vi "Sample Panel.vi"(8 "error in (no error)":errorcluster, 9 "L_Or_R":string, 10 "Measure_No":i64, 11 "connection reference":T1) -> (0 "error out":errorcluster)   [LabVIEW 2015, in "Sample.lvlib"]
uses:
  Sample.lvlib
  <vilib>/userdefined/High Color/IMAQdx.ctl
  Sub VIs/DAQ/DAQ.lvlib
  Sub VIs/CCD/CCD.lvlib
  Sub VIs/Database Processing/Database Processing.lvlib
  <vilib>/addons/database/NI_Database_API.lvlib
  <vilib>/addons/database/_DB Variant To Data/Database Variant To Data.xnode
  Sub VIs/Database Processing/Support/Table/Biometry.ctl
  support/User Event - Stop/User Event - Stop.lvlib
  support/Message Queue/Message Queue.lvlib
  support/Message Queue/Enqueue Message (Single).vi
  Sub VIs/DAQ/DAQ Configuration.ctl
  Sub VIs/CCD/Support/CCD Configuration.ctl
  Support/Sample Configuration.ctl
  <vilib>/Analysis/3filter.llb/Filter Passband Type.ctl
  <vilib>/Analysis/NI_AALBase.lvlib
  <vilib>/Analysis/4window.llb/windowTd.ctl
  <vilib>/Analysis/NI_AALPro.lvlib
  Sub VIs/Digital Signal Processing/Support/DSP Configuration.ctl
  Sub VIs/Digital Signal Processing/Digital Signal Processing.lvlib
  <vilib>/vision/Image Controls.llb/IMAQ Image.ctl
  <vilib>/addons/database/Connection.llb/Conn ObjectReference.ctl
panel:
  in  "Sample":bool
  out "Asan Signal":dbl[](graph)
  in  "停止":bool
  out "CCD Image":T2(plugin-control)
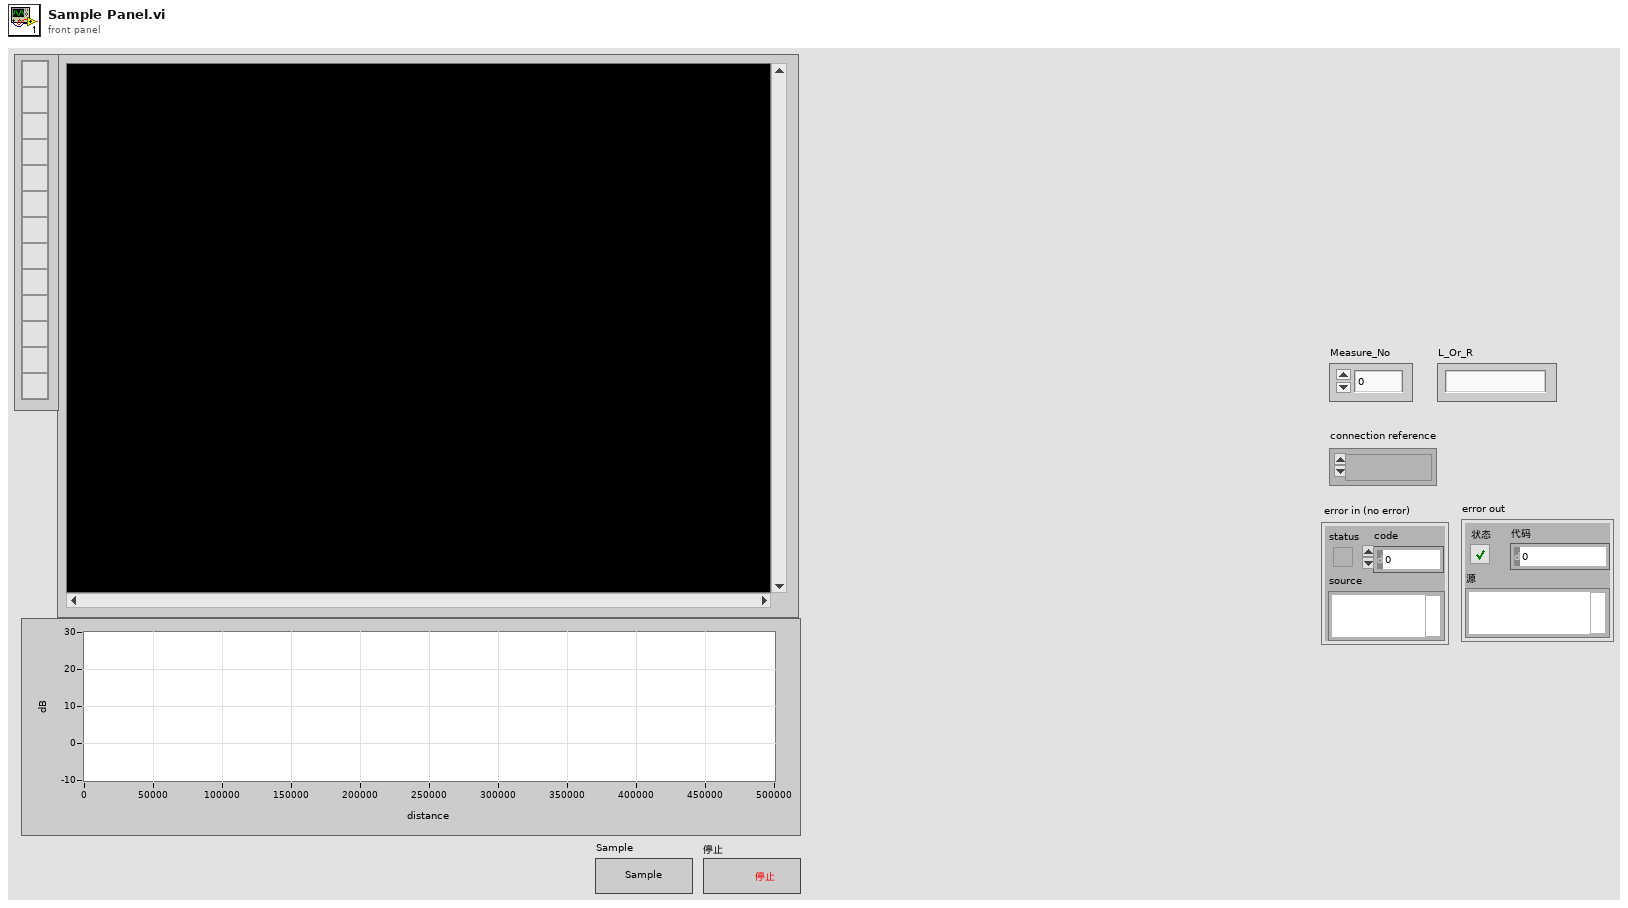
[diagram p1: front panel]
types:
  T1 = typedef "NI_Database_API.lvlib/Conn ObjectReference.ctl" = refnum<k1>
  T2 = typedef "IMAQ Image.ctl" = refnum<image>
  T3 = typedef "Biometry.ctl" = cluster{"Measure_ID":i64, "Measure_No":i64, "Ordinal":i64, "L_Or_R":string, "CCT":sgl, "CCT__State":string, "ACD":sgl, "ACD__State":string, "LT":sgl, "LT__State":string, "RT":sgl, "RT__State":string, "AL":sgl, "AL__State":string, "PD":sgl, "PD__State":string, "PCX":sgl, "PCY":sgl, "WTW":sgl, "WTW__State":string, "ICX":sgl, "ICY":sgl, "K_flat":sgl, "K_steep":sgl, "K_AST":sgl, "K__State":string, "Ascan_data_Original":string, "picture_pupil_Original":string, "picture_WTW_Original":string, "Ascan_data_Processing":string, "picture_pupil_Processing":string, "picture_WTW_Processing":string, "picture_Processing_K":string, "picture_Processing_ALL":string}
  T4 = typedef "Digital Signal Processing.lvlib/DSP Configuration.ctl" = cluster{"Sampling Frequency":dbl, "filter type":T5, "RF Filter Low Frequency":dbl, "RF Filter High Frequency":dbl, "RF Filter Taps":i32, "window":T6, "RF window parameter":dbl, "filter type 2":T5, "Demodulated Filter Low Frequency":dbl, "Demodulated Filter HighFrequency":dbl, "Demodulated Filter Order":i32, "SPAN":i32, "Logarithmic Base":dbl, "Noise path":string, "Work position parameter":i32[]}
  T5 = typedef "NI_AALBase.lvlib/Filter Passband Type.ctl" = enum32{"Lowpass", "Highpass", "Bandpass", "Bandstop"}
  T6 = typedef "NI_AALPro.lvlib/windowTd.ctl" = u32
  T7 = typedef "Sample.lvlib/Sample Configuration.ctl" = cluster{"DAQ Configuration":T8, "CCD Configuration":T9, "DSP Parameter":T4}
  T8 = typedef "DAQ.lvlib/DAQ Configuration.ctl" = cluster{"hDevice":i32, "DevNum":u8, "Configuration Parameter":i32[], "READ_MAX_LEN":i32, "DO":bool[]}
  T9 = typedef "CCD.lvlib/CCD Configuration.ctl" = cluster{"Session In":T10, "New Image":T2}
  T10 = typedef "IMAQdx.ctl" = refnum<k21>
  T11 = typedef "Message Queue.lvlib/All Message Queues Sample Panel.ctl" = cluster{"UI":refnum<queue>, "CAM":refnum<queue>, "CAM Log":refnum<queue>, "DAQ":refnum<queue>, "DSP":refnum<queue>, "DAQ Log":refnum<queue>, "DAQ Read Digital":refnum<queue>}
  T12 = cluster{"filter structure":enum32{"IIR 2nd Order", "IIR 4th Order"}, "Reverse Coefficients":dbl[], "Forward Coefficients":dbl[]}
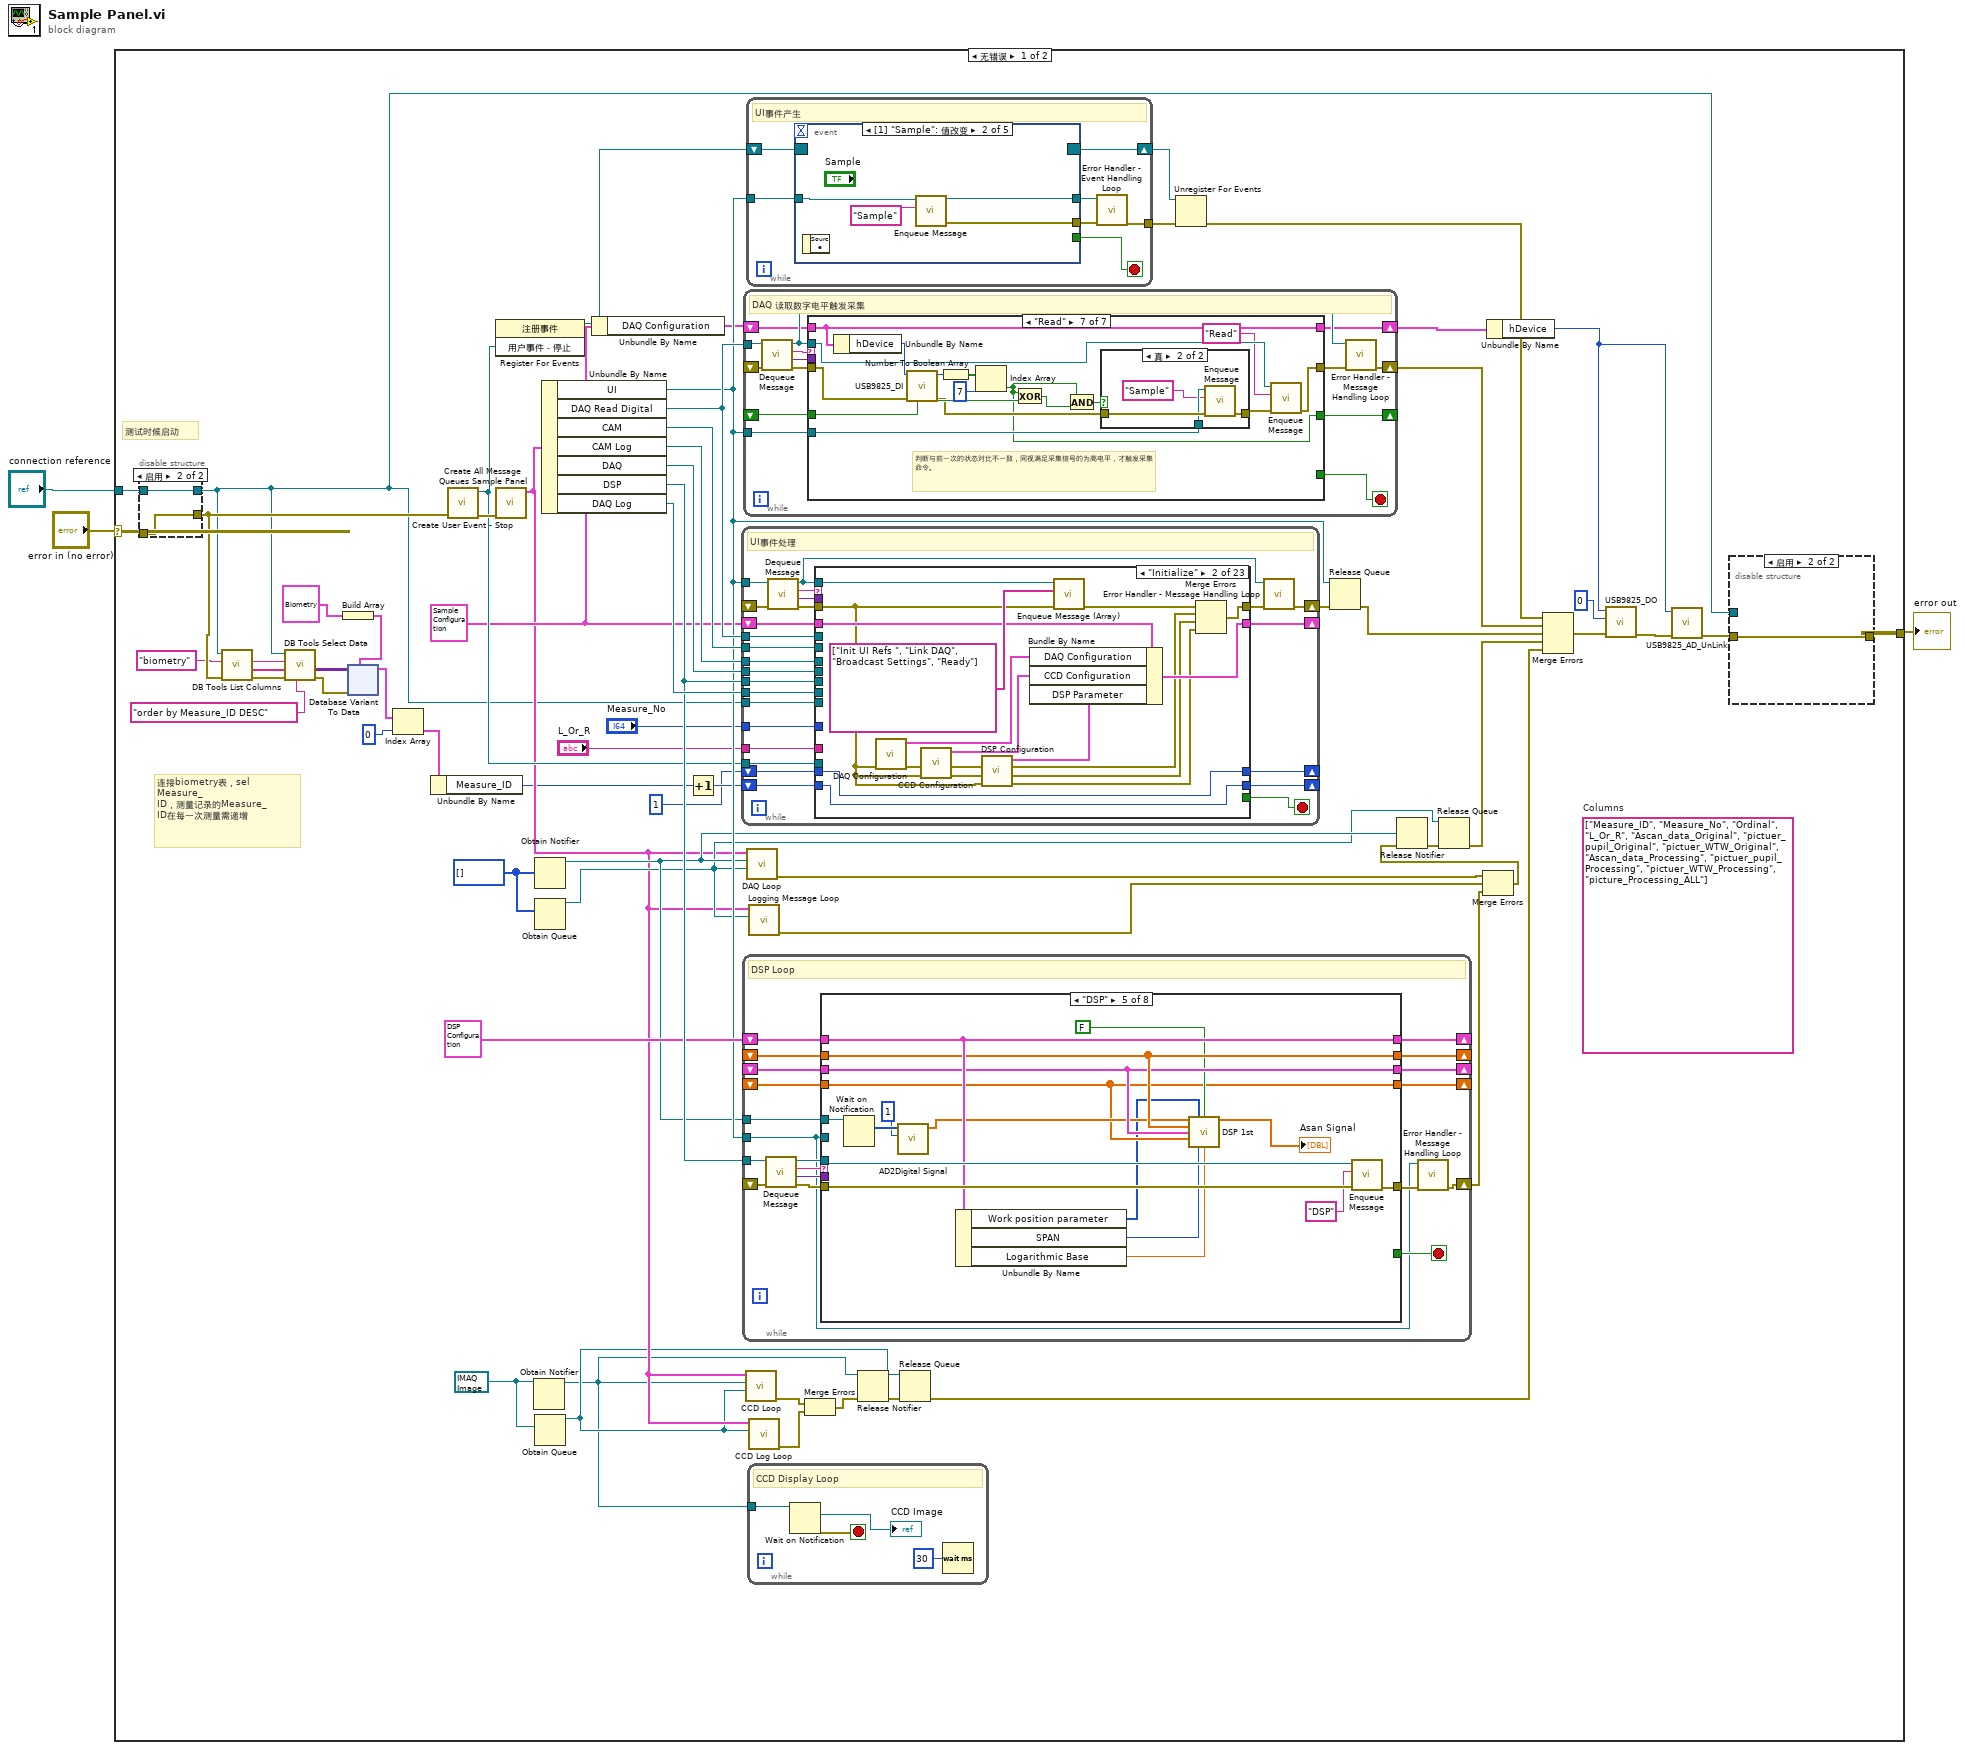
[diagram p0: block diagram]
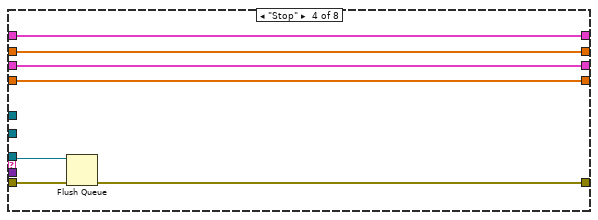
[diagram p5: hidden frame]
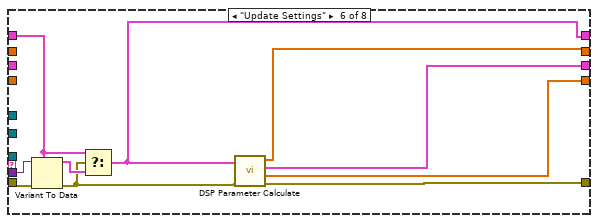
[diagram p6: hidden frame]
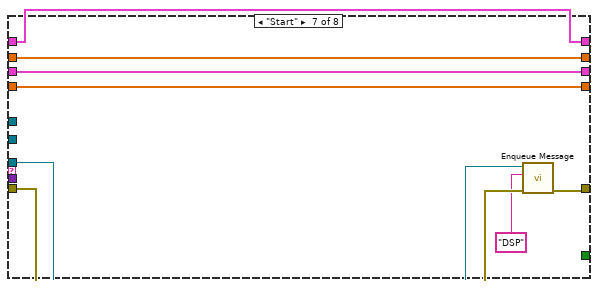
[diagram p7: hidden frame]
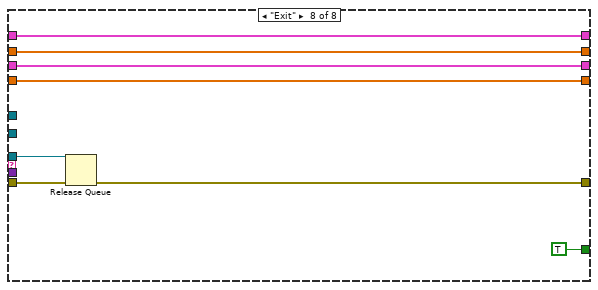
[diagram p8: hidden frame]
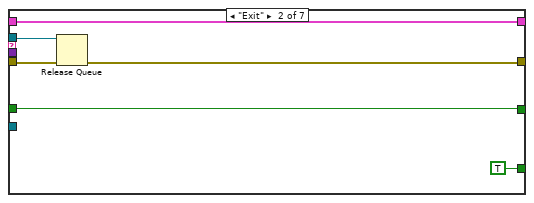
[diagram p10: hidden frame]
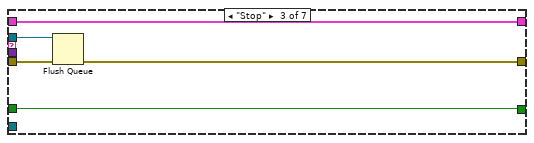
[diagram p11: hidden frame]
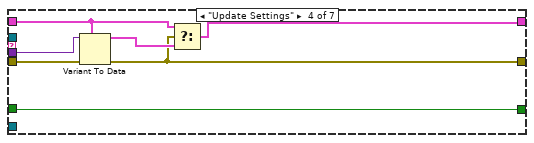
[diagram p12: hidden frame]
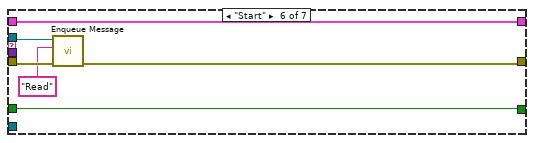
[diagram p14: hidden frame]
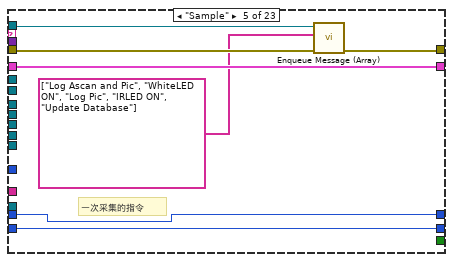
[diagram p19: hidden frame]
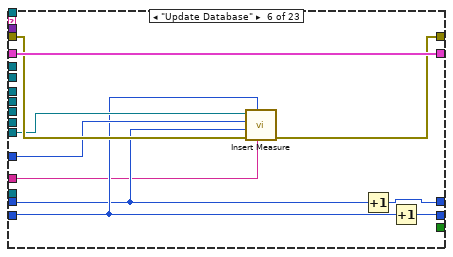
[diagram p20: hidden frame]
diagram:
  n1 = case shown="无错误" "error in (no error)" {
    selector: "error in (no error)" -> [w66 w1567]
    tunnel: "connection reference" -> [w65 _]
    tunnel: [w64 w1567] -> w1
    frame No Error {
      w19 = "biometry" ("table")
      w50 = T2 refnum ("Image Out")
      w53 = i16[] []
      w36 = T7 {"DAQ Configuration"={"hDevice"=0, "DevNum"=0, "Configuration Parameter"=[], "READ_MAX_LEN"=0, "DO"=[]}, "CCD Configuration"={"Session In"="", "New Image"=refnum}, "DSP Parameter"={"Sampling Frequency"=0.0, "filter type"=enum."Lowpass", "RF Filter Low Frequency"=0.0, "RF Filter High Frequency"=0.0, "RF Filter Taps"=0, "window"=0, "RF window parameter"=nan, "filter type 2"=enum."Lowpass", "Demodulated Filter Low Frequency"=0.0, "Demodulated Filter HighFrequency"=0.0, "Demodulated Filter Order"=0, "SPAN"=0, "Logarithmic Base"=0.0, "Noise path"="", "Work position parameter"=[]}} ("Sample Configuration")
      (unwired) string[] ["Measure_ID", "Measure_No", "Ordinal", "L_Or_R", "Ascan_data_Original", "pictuer_pupil_Original", "pictuer_WTW_Original", "Ascan_data_Processing", "pictuer_pupil_Processing", "pictuer_WTW_Processing", "picture_Processing_ALL"]  # Columns
      # "连接biometry表，sel Measure_ID，测量记录的Measure_ID在每一次测量需递增"
      # "测试时候启动"
      n2 = disable-structure shown="启用" {
        disable-tunnel: [w1564 w1565] -> w61
        disable-tunnel: w66 -> [w1563 w1565]
        disable-tunnel: [w1562 w1566] -> w6
        disable-tunnel: w65 -> [_ w1566]
        frame Disabled {
          n3 = call "Connect Database.vi"("error in (no error)"=w1563) -> ("error out"=w1564:errorcluster, "connection reference"=w1562:T1)  [unwired: 9 in]
        }
        frame Enabled {
        }
      }
      n4 = call <vilib>:"DB Tools List Columns.vi"("error in (no error)"=w61, "table"=w19, "connection reference"=w6) -> ("error out"=w17:errorcluster, "columns"=w18:string[])  [unwired: 1 in, 2 out]
      n5 = call <vilib>:"DB Tools Select Data.vi"("condition"="order by Measure_ID DESC", "error in (no error)"=w17, "columns"=w18, "table"=w19, "connection reference"=w6) -> ("error out"=w16:errorcluster, "data"=w15:variant[][])  [unwired: 1 in, 1 out]
      n6 = Build Array(T3 {"Measure_ID"=0, "Measure_No"=0, "Ordinal"=0, "L_Or_R"="", "CCT"=0.0, "CCT__State"="", "ACD"=0.0, "ACD__State"="", "LT"=0.0, "LT__State"="", "RT"=0.0, "RT__State"="", "AL"=0.0, "AL__State"="", "PD"=0.0, "PD__State"="", "PCX"=0.0, "PCY"=0.0, "WTW"=0.0, "WTW__State"="", "ICX"=0.0, "ICY"=0.0, "K_flat"=0.0, "K_steep"=0.0, "K_AST"=0.0, "K__State"="", "Ascan_data_Original"="", "picture_pupil_Original"="", "picture_WTW_Original"="", "Ascan_data_Processing"="", "picture_pupil_Processing"="", "picture_WTW_Processing"="", "picture_Processing_K"="", "picture_Processing_ALL"=""} ("biometry")) -> (w12:T3[])
      n7 = xnode "Database Variant To Data"("database variant"=w15, "error in (no error)"=w16, "type"=w12) -> ("data"=w11:T3[])  [unwired: 1 out]
      n8 = Index Array(array=w11, index=0 ("索引")) -> (element=w10:T3)
      n9 = Unbundle By Name(w10) -> ("Measure_ID"=w8:i64)
      n10 = call "Create User Event - Stop.vi"("error in (no error)"=w61) -> ("error out"=w60:cluster{"状态":bool, "代码":i32, "源":string}, "用户事件－停止"=w37:refnum<user-event>)  [unwired: 9 in]
      n11 = register-events(w37) -> (reference out=w59:refnum<event-registration>)  [unwired: 2 in, 1 out]
      n12 = call "Create All Message Queues Sample Panel.vi"("error in (no error)"=w60) -> ("消息队列"=w25:T11)  [unwired: 9 in, 1 out]
      n13 = Obtain Notifier(notification data type=w50) -> (notifier out=w20:refnum<notifier>)  [unwired: 3 in, 2 out]
      n14 = Obtain Notifier(notification data type=w53) -> (notifier out=w39:refnum<notifier>)  [unwired: 3 in, 2 out]
      n15 = Obtain Queue(element data type=w53) -> (queue out=w29:refnum<queue>)  [unwired: 4 in, 2 out]
      n16 = Obtain Queue(element data type=w50) -> (queue out=w21:refnum<queue>)  [unwired: 4 in, 2 out]
      n17 = Unbundle By Name(w25) -> ("UI"=w41:refnum<queue>, "DAQ Read Digital"=w58:refnum<queue>, "CAM"=w57:refnum<queue>, "CAM Log"=w56:refnum<queue>, "DAQ"=w55:refnum<queue>, "DSP"=w52:refnum<queue>, "DAQ Log"=w54:refnum<queue>)
      n18 = Unbundle By Name(w36) -> ("DAQ Configuration"=w35:T8)
      n19 = Increment(x=w8) -> (x+1=w26:i64)
      n20 = while {
        tunnel: w41 -> [w1309]
        shift-right: [w1304] -> w42
        shift-left: _ -> [w1306]
        shift-right: [w1301] -> _
        shift-left: w36 -> [w1302]
        tunnel: w58 -> [w1300]
        tunnel: w57 -> [w1299]
        tunnel: w56 -> [w1298]
        tunnel: w55 -> [w1297]
        tunnel: w52 -> [w1296]
        tunnel: w54 -> [w1295]
        tunnel: w37 -> [w1292]
        shift-right: [w1290] -> _
        shift-left: w26 -> [w1291]
        shift-right: [w1288] -> _
        shift-left: 1 -> [w1289]
        tunnel: w6 -> [w1287]
        tunnel: "Measure_No" -> [w1286]
        tunnel: "L_Or_R" -> [w1285]
        stop <- w1293 stop-if-true
        # "UI事件处理"
        n21 = call "Dequeue Message.vi"("error in (no error)"=w1306, "消息队列"=w1309) -> ("error out"=w1307:cluster{"状态":bool, "代码":i32, "源":string}, "消息数据"=w1294:variant, "消息"=w1308:string, "消息队列副本"=w1303:refnum<queue>)  [unwired: 6 in]
        n22 = case shown="\"Initialize\"" w1308 {
          tunnel: w1303 -> [_ w1328 _ _ w1339 _ _ _ _ w1386 _ _ _ _ _ _ _ _ _ w1477 _ _ _]
          tunnel: w1307 -> [w1313 w1316 w1331 w1335 w1341 w1350 w1365 w1369 w1379 w1390 w1399 w1408 w1417 w1426 w1433 w1451 w1460 w1463 w1469 w1479 w1496 w1514 w1535]
          tunnel: [w1313 w1322 w1331 w1335 w1340 w1349 w1356 w1368 w1378 w1387 w1395 w1404 w1413 w1422 w1432 w1442 w1459 w1463 w1468 w1478 w1489 w1501 w1520] -> w1305
          tunnel: w1302 -> [w1312 w1326 w1332 w1336 w1343 w1353 w1363 w1374 w1383 w1391 w1402 w1411 w1420 w1429 w1436 w1452 w1458 w1464 w1472 w1480 w1497 w1515 w1536]
          tunnel: [w1312 w1323 w1332 w1336 w1343 w1353 w1363 w1374 w1383 w1391 w1402 w1411 w1420 w1429 w1436 w1452 w1455 w1464 w1472 w1480 w1497 w1515 w1536] -> w1301
          tunnel: w1300 -> [_ _ _ _ _ _ _ _ _ _ _ _ _ _ _ w1449 _ _ _ _ w1495 w1513 w1534]
          tunnel: w1299 -> [_ _ _ _ _ _ _ _ _ _ _ _ _ _ _ w1446 _ _ _ _ w1488 w1507 w1528]
          tunnel: w1298 -> [_ _ _ _ _ _ w1361 w1373 _ _ _ _ _ _ _ _ _ _ _ _ w1487 w1506 w1527]
          tunnel: w1297 -> [_ _ _ _ _ _ _ _ _ _ _ _ _ _ _ w1448 _ _ _ _ w1486 w1505 w1526]
          tunnel: w1296 -> [_ _ _ _ _ _ _ _ _ _ _ _ _ _ _ w1441 _ _ _ _ w1485 w1504 w1525]
          tunnel: w1295 -> [_ _ _ _ _ _ w1364 _ w1377 _ _ _ _ _ _ _ _ _ _ _ w1484 w1503 w1524]
          tunnel: w1294 -> [_ _ _ _ _ _ _ _ _ _ _ _ _ _ _ _ _ _ w1467 _ _ _ _]
          tunnel: [_ _ _ _ _ _ _ _ _ _ _ _ _ _ _ _ _ _ _ _ _ _ TRUE] -> w1293
          tunnel: w1292 -> [_ _ _ _ _ _ _ _ _ _ _ _ _ _ _ _ _ _ _ _ _ _ w1518]
          tunnel: w1291 -> [w1311 w1315 w1330 w1334 w1342 w1346 w1355 w1367 w1376 w1389 w1398 w1407 w1416 w1425 w1431 w1438 w1454 w1462 w1466 w1474 w1482 w1500 w1517]
          tunnel: [w1311 w1315 w1330 w1334 w1342 w1352 w1355 w1367 w1376 w1389 w1398 w1407 w1416 w1425 w1431 w1438 w1454 w1462 w1466 w1474 w1482 w1500 w1517] -> w1290
          tunnel: w1289 -> [w1310 w1314 w1329 w1333 w1337 w1345 w1354 w1366 w1375 w1384 w1394 w1403 w1412 w1421 w1430 w1437 w1453 w1461 w1465 w1473 w1481 w1498 w1516]
          tunnel: [w1310 w1314 w1329 w1333 w1337 w1351 w1354 w1366 w1375 w1384 w1394 w1403 w1412 w1421 w1430 w1437 w1453 w1461 w1465 w1473 w1481 w1498 w1516] -> w1288
          tunnel: w1287 -> [_ _ _ _ _ w1348 _ _ _ _ _ _ _ _ _ _ _ _ _ _ _ _ _]
          tunnel: w1286 -> [_ _ _ _ _ w1347 _ _ _ _ _ _ _ _ _ _ _ _ _ _ _ _ _]
          tunnel: w1285 -> [_ _ _ _ _ w1344 _ _ _ _ _ _ _ _ _ _ _ _ _ _ _ _ _]
          frame Default {
          }
          frame "Initialize" {
            n23 = call "DAQ Configuration.vi"("error in (no error)"=w1316) -> ("error out"=w1320:errorcluster, "parameter output"=w1325:T8)  [unwired: 9 in]
            n24 = call "CCD Configuration.vi"("error in (no error)"=w1316) -> ("error out"=w1318:errorcluster, "CCD Configuration"=w1324:T9)  [unwired: 9 in]
            n25 = call "DSP Configuration.vi"("error in (no error)"=w1316) -> ("error out"=w1317:errorcluster, "DSP Parameter Output"=w1319:T4)  [unwired: 9 in]
            n26 = Bundle By Name(cluster=w1326, "DAQ Configuration"=w1325, "CCD Configuration"=w1324, "DSP Parameter"=w1319) -> (w1323:T7)
            n27 = call "Enqueue Message (Array).vi"("error in (no error)"=w1316, "消息数组"=string[] ["Init UI Refs ", "Link DAQ", "Broadcast Settings", "Ready"], "消息队列"=w1328) -> ("error out"=w1321:cluster{"状态":bool, "代码":i32, "源":string})  [unwired: 7 in, 1 out]
            n28 = Merge Errors(w1321, w1320, w1318, w1317) -> (w1322:errorcluster)
          }
          frame "Init UI Refs" {
          }
          frame "Copy this frame" {
          }
          frame "Sample" {
            # "一次采集的指令"
            n29 = call "Enqueue Message (Array).vi"("error in (no error)"=w1341, "消息数组"=string[] ["Log Ascan and Pic", "WhiteLED ON", "Log Pic", "IRLED ON", "Update Database"], "消息队列"=w1339) -> ("error out"=w1340:cluster{"状态":bool, "代码":i32, "源":string})  [unwired: 7 in, 1 out]
          }
          frame "Update Database" {
            n30 = call "Insert Measure.vi"("Left Or Right"=w1344, "Measure_ID"=w1346, "Error In"=w1350, "Ordinal"=w1345, "Measure_No"=w1347, "connection reference"=w1348) -> ("Error Out"=w1349:errorcluster)  [unwired: 5 in]
            n31 = Increment(x=w1345) -> (x+1=w1351:i32)
            n32 = Increment(x=w1346) -> (x+1=w1352:i64)
          }
          frame "Log Ascan and Pic" {
            n33 = call-poly "Enqueue Message.vi"("error in (no error)"=w1365, "消息数据"=w1355, "消息"="Save", "消息队列"=w1364) -> ("error out"=w1362:cluster{"状态":bool, "代码":i32, "源":string})  [unwired: 6 in, 1 out]
            n34 = call-poly "Enqueue Message.vi"("error in (no error)"=w1362, "消息数据"=w1355, "消息"="SaveIR", "消息队列"=w1361) -> ("error out"=w1358:cluster{"状态":bool, "代码":i32, "源":string})  [unwired: 6 in, 1 out]
            n35 = call "时间延迟5"("error in (no error)"=w1358, "Delay Time (s)"=0.5) -> ("error out"=w1356:errorcluster)  [unwired: 9 in]
          }
          frame "Log Pic" {
            n36 = call-poly "Enqueue Message.vi"("error in (no error)"=w1369, "消息数据"=w1367, "消息"="SaveWTW", "消息队列"=w1373) -> ("error out"=w1371:cluster{"状态":bool, "代码":i32, "源":string})  [unwired: 6 in, 1 out]
            n37 = call "时间延迟6"("error in (no error)"=w1371, "Delay Time (s)"=0.5) -> ("error out"=w1368:errorcluster)  [unwired: 9 in]
          }
          frame "Log Ascan" {
            n38 = call-poly "Enqueue Message.vi"("error in (no error)"=w1379, "消息数据"=w1376, "消息"="Save", "消息队列"=w1377) -> ("error out"=w1381:cluster{"状态":bool, "代码":i32, "源":string})  [unwired: 6 in, 1 out]
            n39 = call "时间延迟7"("error in (no error)"=w1381, "Delay Time (s)"=0.5) -> ("error out"=w1378:errorcluster)  [unwired: 9 in]
          }
          frame "Ready" {
            # "开启仪器的步骤指令"
            n40 = flat-sequence {
              tunnel: [w1392] -> w1388
              tunnel: w1390 -> [w1392]
              frame #0 {
                n41 = One Button Dialog(message="点击开启" ("消息")) -> ()  [unwired: 1 in, 1 out]
              }
            }
            n42 = call "Enqueue Message (Array).vi"("error in (no error)"=w1388, "消息数组"=string[] ["SLD ON", "MOTOR ON", "IRLED ON", "Start"], "消息队列"=w1386) -> ("error out"=w1387:cluster{"状态":bool, "代码":i32, "源":string})  [unwired: 7 in, 1 out]
          }
          frame "SLD ON" {
            n43 = Unbundle By Name(w1402) -> ("DAQ Configuration.hDevice"=w1401:i32)
            n44 = call "USB9825_DO.vi"("Error In"=w1399, "pDO"=u8 8, "hDevice"=w1401) -> ("Error Out"=w1397:errorcluster)  [unwired: 8 in]
            n45 = call "时间延迟"("error in (no error)"=w1397, "Delay Time (s)"=0.01) -> ("error out"=w1395:errorcluster)  [unwired: 9 in]
          }
          frame "MOTOR ON" {
            # "开启电机，同时保留SLD开启。"
            n46 = Unbundle By Name(w1411) -> ("DAQ Configuration.hDevice"=w1410:i32)
            n47 = call "USB9825_DO.vi"("Error In"=w1408, "pDO"=u8 24, "hDevice"=w1410) -> ("Error Out"=w1406:errorcluster)  [unwired: 8 in]
            n48 = call "时间延迟2"("error in (no error)"=w1406, "Delay Time (s)"=0.01) -> ("error out"=w1404:errorcluster)  [unwired: 9 in]
          }
          frame "IRLED ON" {
            # "开启IRLED，同时保留电机和SLD开启。"
            n49 = Unbundle By Name(w1420) -> ("DAQ Configuration.hDevice"=w1419:i32)
            n50 = call "USB9825_DO.vi"("Error In"=w1417, "pDO"=u8 216, "hDevice"=w1419) -> ("Error Out"=w1415:errorcluster)  [unwired: 8 in]
            n51 = call "时间延迟3"("error in (no error)"=w1415, "Delay Time (s)"=0.01) -> ("error out"=w1413:errorcluster)  [unwired: 9 in]
          }
          frame "WhiteLED ON" {
            # "开启白光LED，同时保留电机和SLD开启。"
            n52 = Unbundle By Name(w1429) -> ("DAQ Configuration.hDevice"=w1428:i32)
            n53 = call "USB9825_DO.vi"("Error In"=w1426, "pDO"=u8 56, "hDevice"=w1428) -> ("Error Out"=w1424:errorcluster)  [unwired: 8 in]
            n54 = call "时间延迟4"("error in (no error)"=w1424, "Delay Time (s)"=0.5) -> ("error out"=w1422:errorcluster)  [unwired: 9 in]
          }
          frame "OFF" {
            # "216是开启SLD、电机和红外LED。"
            n55 = Unbundle By Name(w1436) -> ("DAQ Configuration.hDevice"=w1435:i32)
            n56 = call "USB9825_DO.vi"("Error In"=w1433, "pDO"=u8 0, "hDevice"=w1435) -> ("Error Out"=w1432:errorcluster)  [unwired: 8 in]
          }
          frame "Broadcast Settings" {
            w1440 = "Update Settings" ("消息")
            # "推送设置到DAQ读取数字电平、DAQ和相机采集循环。"
            n57 = Unbundle By Name(w1452) -> ("DAQ Configuration"=w1445:T8, "CCD Configuration"=w1444:T9, "DSP Parameter"=w1439:T4)
            n58 = call-poly "Enqueue Message.vi"("error in (no error)"=w1451, "消息数据"=w1445, "消息"=w1440, "消息队列"=w1449) -> ("error out"=w1450:cluster{"状态":bool, "代码":i32, "源":string})  [unwired: 6 in, 1 out]
            n59 = call-poly "Enqueue Message.vi"("error in (no error)"=w1450, "消息数据"=w1445, "消息"=w1440, "消息队列"=w1448) -> ("error out"=w1447:cluster{"状态":bool, "代码":i32, "源":string})  [unwired: 6 in, 1 out]
            n60 = call-poly "Enqueue Message.vi"("error in (no error)"=w1447, "消息数据"=w1444, "消息"=w1440, "消息队列"=w1446) -> ("error out"=w1443:cluster{"状态":bool, "代码":i32, "源":string})  [unwired: 6 in, 1 out]
            n61 = call-poly "Enqueue Message.vi"("error in (no error)"=w1443, "消息数据"=w1439, "消息"=w1440, "消息队列"=w1441) -> ("error out"=w1442:cluster{"状态":bool, "代码":i32, "源":string})  [unwired: 6 in, 1 out]
          }
          frame "Link DAQ" {
            n62 = call "USB9825_AD_Link.vi"("Error In"=w1460) -> ("Error Out"=w1459:errorcluster, "DevNum"=w1456:i32, "hDevice"=w1457:i32)  [unwired: 7 in, 1 out]
            n63 = Bundle By Name(cluster=w1458, "DAQ Configuration.hDevice"=w1457, "DAQ Configuration.DevNum"=w1456) -> (w1455:T7)
          }
          frame "Update State" {
          }
          frame "Error" {
            n64 = Variant To Data(error in=w1469, type=errorcluster {"status"=FALSE, "code"=0, "source"=""} ("error constant"), Variant=w1467) -> (data=w1470:errorcluster, error out=w1468:errorcluster)
            n65 = call <vilib>:"Simple Error Handler.vi"("error in (no error)"=w1470) -> ()  [unwired: 4 in, 5 out]
          }
          frame "Confirm Quit" {
            n66 = call-poly "Enqueue Message.vi"("优先消息？ (F)"=TRUE, "error in (no error)"=w1479, "消息"="Exit", "消息队列"=w1477) -> ("error out"=w1478:cluster{"状态":bool, "代码":i32, "源":string})  [unwired: 6 in, 1 out]
          }
          frame "Start" {
            w1483 = "Start" ("消息")
            # "开启DAQ读取数字电平、相机、相机保存、DAQ、DAQ保存循环。"
            n67 = call-poly "Enqueue Message.vi"("error in (no error)"=w1496, "消息"=w1483, "消息队列"=w1495) -> ("error out"=w1494:cluster{"状态":bool, "代码":i32, "源":string})  [unwired: 7 in, 1 out]
            n68 = call-poly "Enqueue Message.vi"("error in (no error)"=w1494, "消息"=w1483, "消息队列"=w1488) -> ("error out"=w1493:cluster{"状态":bool, "代码":i32, "源":string})  [unwired: 7 in, 1 out]
            n69 = call-poly "Enqueue Message.vi"("error in (no error)"=w1493, "消息"=w1483, "消息队列"=w1487) -> ("error out"=w1492:cluster{"状态":bool, "代码":i32, "源":string})  [unwired: 7 in, 1 out]
            n70 = call-poly "Enqueue Message.vi"("error in (no error)"=w1492, "消息"=w1483, "消息队列"=w1486) -> ("error out"=w1491:cluster{"状态":bool, "代码":i32, "源":string})  [unwired: 7 in, 1 out]
            n71 = call-poly "Enqueue Message.vi"("error in (no error)"=w1491, "消息"=w1483, "消息队列"=w1485) -> ("error out"=w1490:cluster{"状态":bool, "代码":i32, "源":string})  [unwired: 7 in, 1 out]
            n72 = call-poly "Enqueue Message.vi"("error in (no error)"=w1490, "消息"=w1483, "消息队列"=w1484) -> ("error out"=w1489:cluster{"状态":bool, "代码":i32, "源":string})  [unwired: 7 in, 1 out]
          }
          frame "Stop" {
            w1499 = TRUE ("优先消息？ (F)")
            w1502 = "Stop" ("消息")
            # "停止DAQ读取数字电平、相机、相机保存、DAQ、DAQ保存循环。"
            n73 = call-poly "Enqueue Message.vi"("优先消息？ (F)"=w1499, "error in (no error)"=w1514, "消息"=w1502, "消息队列"=w1513) -> ("error out"=w1512:cluster{"状态":bool, "代码":i32, "源":string})  [unwired: 6 in, 1 out]
            n74 = call-poly "Enqueue Message.vi"("优先消息？ (F)"=w1499, "error in (no error)"=w1512, "消息"=w1502, "消息队列"=w1507) -> ("error out"=w1511:cluster{"状态":bool, "代码":i32, "源":string})  [unwired: 6 in, 1 out]
            n75 = call-poly "Enqueue Message.vi"("优先消息？ (F)"=w1499, "error in (no error)"=w1511, "消息"=w1502, "消息队列"=w1506) -> ("error out"=w1510:cluster{"状态":bool, "代码":i32, "源":string})  [unwired: 6 in, 1 out]
            n76 = call-poly "Enqueue Message.vi"("优先消息？ (F)"=w1499, "error in (no error)"=w1510, "消息"=w1502, "消息队列"=w1505) -> ("error out"=w1509:cluster{"状态":bool, "代码":i32, "源":string})  [unwired: 6 in, 1 out]
            n77 = call-poly "Enqueue Message.vi"("优先消息？ (F)"=w1499, "error in (no error)"=w1509, "消息"=w1502, "消息队列"=w1504) -> ("error out"=w1508:cluster{"状态":bool, "代码":i32, "源":string})  [unwired: 6 in, 1 out]
            n78 = call-poly "Enqueue Message.vi"("优先消息？ (F)"=w1499, "error in (no error)"=w1508, "消息"=w1502, "消息队列"=w1503) -> ("error out"=w1501:cluster{"状态":bool, "代码":i32, "源":string})  [unwired: 6 in, 1 out]
          }
          frame "Exit" {
            w1522 = TRUE ("优先消息？ (F)")
            w1523 = "Exit" ("消息")
            n79 = call-poly "Enqueue Message.vi"("优先消息？ (F)"=w1522, "error in (no error)"=w1535, "消息"=w1523, "消息队列"=w1534) -> ("error out"=w1533:cluster{"状态":bool, "代码":i32, "源":string})  [unwired: 6 in, 1 out]
            n80 = call-poly "Enqueue Message.vi"("优先消息？ (F)"=w1522, "error in (no error)"=w1533, "消息"=w1523, "消息队列"=w1528) -> ("error out"=w1532:cluster{"状态":bool, "代码":i32, "源":string})  [unwired: 6 in, 1 out]
            n81 = call-poly "Enqueue Message.vi"("优先消息？ (F)"=w1522, "error in (no error)"=w1532, "消息"=w1523, "消息队列"=w1527) -> ("error out"=w1531:cluster{"状态":bool, "代码":i32, "源":string})  [unwired: 6 in, 1 out]
            n82 = call-poly "Enqueue Message.vi"("优先消息？ (F)"=w1522, "error in (no error)"=w1531, "消息"=w1523, "消息队列"=w1526) -> ("error out"=w1530:cluster{"状态":bool, "代码":i32, "源":string})  [unwired: 6 in, 1 out]
            n83 = call-poly "Enqueue Message.vi"("优先消息？ (F)"=w1522, "error in (no error)"=w1530, "消息"=w1523, "消息队列"=w1525) -> ("error out"=w1529:cluster{"状态":bool, "代码":i32, "源":string})  [unwired: 6 in, 1 out]
            n84 = call-poly "Enqueue Message.vi"("优先消息？ (F)"=w1522, "error in (no error)"=w1529, "消息"=w1523, "消息队列"=w1524) -> ("error out"=w1519:cluster{"状态":bool, "代码":i32, "源":string})  [unwired: 6 in, 1 out]
            n85 = call "Fire User Event - Stop.vi"("error in (no error)"=w1519, "用户事件－停止"=w1518) -> ("error out"=w1520:cluster{"状态":bool, "代码":i32, "源":string})  [unwired: 9 in]
          }
        }
        n86 = call "Error Handler - Message Handling Loop.vi"("error in (no error)"=w1305, "消息队列"=w1303) -> ("错误输入副本"=w1304:cluster{"状态":bool, "代码":i32, "源":string})  [unwired: 8 in, 1 out]
      }
      n87 = while {
        tunnel: w52 -> [w1150]
        shift-right: [w1148] -> _
        shift-left: T4 {"Sampling Frequency"=0.0, "filter type"=enum."Lowpass", "RF Filter Low Frequency"=0.0, "RF Filter High Frequency"=0.0, "RF Filter Taps"=0, "window"=0, "RF window parameter"=nan, "filter type 2"=enum."Lowpass", "Demodulated Filter Low Frequency"=0.0, "Demodulated Filter HighFrequency"=0.0, "Demodulated Filter Order"=0, "SPAN"=0, "Logarithmic Base"=0.0, "Noise path"="", "Work position parameter"=[]} ("DSP Parameter") -> [w1147]
        tunnel: w41 -> [w1134]
        shift-right: [w1135] -> w28
        shift-left: _ -> [w1145]
        shift-right: [w1141] -> _
        shift-left: _ -> [w1140]
        shift-right: [w1139] -> _
        shift-left: _ -> [w1138]
        tunnel: w39 -> [w1137]
        shift-right: [w1133] -> _
        shift-left: _ -> [w1132]
        stop <- w1142 stop-if-true
        # "DSP Loop"
        n88 = call "Dequeue Message.vi"("error in (no error)"=w1145, "消息队列"=w1150) -> ("error out"=w1144:cluster{"状态":bool, "代码":i32, "源":string}, "消息数据"=w1146:variant, "消息"=w1149:string, "消息队列副本"=w1143:refnum<queue>)  [unwired: 6 in]
        n89 = case shown="\"DSP\"" w1149 {
          tunnel: [w1154 w1157 w1165 w1172 w1182 w1195 w1207 w1215] -> w1148
          tunnel: w1147 -> [w1154 w1157 w1165 w1172 w1182 w1196 w1207 w1215]
          tunnel: w1146 -> [_ _ _ _ _ w1197 _ _]
          tunnel: [w1155 w1156 w1164 w1168 w1185 w1190 w1205 w1209] -> w1136
          tunnel: w1144 -> [w1155 w1156 w1164 w1169 w1186 w1198 w1206 w1214]
          tunnel: w1134 -> [_ _ _ _ _ _ _ _]
          tunnel: w1143 -> [_ _ _ w1167 w1184 _ w1204 w1213]
          tunnel: [_ _ _ _ _ _ _ TRUE] -> w1142
          tunnel: [w1153 w1160 w1163 w1171 w1180 w1194 w1202 w1211] -> w1141
          tunnel: w1140 -> [w1153 w1160 w1163 w1171 w1180 _ w1202 w1211]
          tunnel: [w1152 w1159 w1162 w1170 w1179 w1193 w1201 w1210] -> w1139
          tunnel: w1138 -> [w1152 w1159 w1162 w1170 w1179 _ w1201 w1210]
          tunnel: w1137 -> [_ _ _ _ w1189 _ _ _]
          tunnel: [w1151 w1158 w1161 w1166 w1174 w1192 w1200 w1208] -> w1133
          tunnel: w1132 -> [w1151 w1158 w1161 w1166 w1174 _ w1200 w1208]
          frame Default {
          }
          frame "Initialize" {
          }
          frame "Copy this frame" {
          }
          frame "Stop" {
            n90 = Flush Queue(queue=w1167, error in (no error)=w1169) -> (error out=w1168:errorcluster)  [unwired: 2 out]
          }
          frame "DSP" {
            n91 = Wait on Notification(notifier=w1189) -> (notification=w1188:i16[])  [unwired: 3 in, 3 out]
            n92 = call "AD2Digital Signal.vi"("通道数"=1, "AD"=w1188) -> ("CH1"=w1178:dbl[])  [unwired: 8 in, 1 out]
            n93 = Unbundle By Name(w1182) -> ("Work position parameter"=w1173:i32[], "SPAN"=w1177:i32, "Logarithmic Base"=w1176:dbl)
            n94 = call "DSP 1st.vi"("Input Signal"=w1178, "Work position parameter"=w1173, "Minus Noise(F : Don't)"=FALSE, "RF Window"=w1180, "IIR Filter Cluster"=w1179, "Noise Signal"=w1174, "SPAN"=w1177, "Logarithmic Base"=w1176) -> ("DSP signal"=→"Asan Signal":dbl[])  [unwired: 6 in, 1 out]
            n95 = call-poly "Enqueue Message.vi"("error in (no error)"=w1186, "消息"="DSP", "消息队列"=w1184) -> ("error out"=w1185:cluster{"状态":bool, "代码":i32, "源":string})  [unwired: 7 in, 1 out]
          }
          frame "Update Settings" {
            n96 = Variant To Data(error in=w1198, type=w1196, Variant=w1197) -> (data=w1199:T4, error out=w1191:errorcluster)
            n97 = Select(t=w1196, s=w1191, f=w1199) -> (s? t:f=w1195:T4)
            n98 = call "DSP Parameter Calculate.vi"("error in (no error)"=w1191, "DSP Parameter"=w1195) -> ("error out"=w1190:errorcluster, "Noise"=w1192:dbl[], "IIR Filter Cluster"=w1193:T12, "FIR Windowed Coefficients"=w1194:dbl[])  [unwired: 4 in, 2 out]
          }
          frame "Start" {
            n99 = call-poly "Enqueue Message.vi"("error in (no error)"=w1206, "消息"="DSP", "消息队列"=w1204) -> ("error out"=w1205:cluster{"状态":bool, "代码":i32, "源":string})  [unwired: 7 in, 1 out]
          }
          frame "Exit" {
            n100 = Release Queue(queue=w1213, error in (no error)=w1214) -> (error out=w1209:errorcluster)  [unwired: 1 in, 2 out]
          }
        }
        n101 = call "Error Handler - Message Handling Loop.vi"("error in (no error)"=w1136, "消息队列"=w1134) -> ("错误输入副本"=w1135:cluster{"状态":bool, "代码":i32, "源":string})  [unwired: 8 in, 1 out]
      }
      n102 = while {
        tunnel: w58 -> [w1233]
        shift-right: [w1228] -> w45
        shift-left: _ -> [w1230]
        shift-right: [w1222] -> w49
        shift-left: w35 -> [w1226]
        shift-right: [w1225] -> _
        shift-left: _ -> [w1224]
        tunnel: w41 -> [w1223]
        stop <- w1220 stop-if-true
        # "DAQ 读取数字电平触发采集"
        n103 = call "Dequeue Message.vi"("error in (no error)"=w1230, "消息队列"=w1233) -> ("error out"=w1231:cluster{"状态":bool, "代码":i32, "源":string}, "消息数据"=w1221:variant, "消息"=w1232:string, "消息队列副本"=w1227:refnum<queue>)  [unwired: 6 in]
        n104 = case shown="\"Read\"" w1232 {
          tunnel: w1227 -> [_ w1238 w1243 _ _ w1262 w1266]
          tunnel: w1231 -> [w1236 w1240 w1245 w1254 w1257 w1263 w1279]
          tunnel: [w1236 w1239 w1244 w1249 w1257 w1261 w1267] -> w1229
          tunnel: w1226 -> [w1234 w1241 w1246 w1251 w1256 w1258 w1264]
          tunnel: [w1235 w1242 w1247 w1248 w1255 w1259 w1269] -> w1225
          tunnel: w1224 -> [w1235 w1242 w1247 w1248 w1255 w1259 w1274]
          tunnel: w1223 -> [_ _ _ _ _ _ w1272]
          tunnel: [w1234 w1241 w1246 w1250 w1256 w1258 w1264] -> w1222
          tunnel: w1221 -> [_ _ _ w1253 _ _ _]
          tunnel: [_ TRUE _ _ _ _ _] -> w1220
          frame Default {
          }
          frame "Exit" {
            n105 = Release Queue(queue=w1238, error in (no error)=w1240) -> (error out=w1239:errorcluster)  [unwired: 1 in, 2 out]
          }
          frame "Stop" {
            n106 = Flush Queue(queue=w1243, error in (no error)=w1245) -> (error out=w1244:errorcluster)  [unwired: 2 out]
          }
          frame "Update Settings" {
            n107 = Variant To Data(error in=w1254, type=w1251, Variant=w1253) -> (data=w1252:T8, error out=w1249:errorcluster)
            n108 = Select(t=w1251, s=w1249, f=w1252) -> (s? t:f=w1250:T8)
          }
          frame "initialize" {
          }
          frame "Start" {
            n109 = call-poly "Enqueue Message.vi"("error in (no error)"=w1263, "消息"="Read", "消息队列"=w1262) -> ("error out"=w1261:cluster{"状态":bool, "代码":i32, "源":string})  [unwired: 7 in, 1 out]
          }
          frame "Read" {
            # "判断与前一次的状态对比不一致，同视满足采集信号的为高电平，才触发采集命令。"
            n110 = Unbundle By Name(w1264) -> ("hDevice"=w1278:i32)
            n111 = call "USB9825_DI.vi"("错误输入（无错误）"=w1279, "hDevice"=w1278) -> ("错误输出"=w1273:errorcluster, "pDI"=w1277:u8)  [unwired: 8 in]
            n112 = Number To Boolean Array(number=w1277) -> (Boolean array=w1276:bool[])
            n113 = Index Array(array=w1276, index=7 ("索引")) -> (element=w1269:bool)
            n114 = Exclusive Or(1:w1274, 2:w1269) -> (0:w1270:bool)
            n115 = And(x=w1269, y=w1270) -> (x .and. y?=w1271:bool)
            n116 = case shown="真" w1271 {
              tunnel: w1273 -> [w1280 w1284]
              tunnel: [w1280 w1283] -> w1268
              tunnel: w1272 -> [_ w1282]
              frame False {
              }
              frame True {
                n117 = call-poly "Enqueue Message.vi"("error in (no error)"=w1284, "消息"="Sample", "消息队列"=w1282) -> ("error out"=w1283:cluster{"状态":bool, "代码":i32, "源":string})  [unwired: 7 in, 1 out]
              }
            }
            n118 = call-poly "Enqueue Message.vi"("error in (no error)"=w1268, "消息"="Read", "消息队列"=w1266) -> ("error out"=w1267:cluster{"状态":bool, "代码":i32, "源":string})  [unwired: 7 in, 1 out]
          }
        }
        n119 = call "Error Handler - Message Handling Loop.vi"("error in (no error)"=w1229, "消息队列"=w1227) -> ("错误输入副本"=w1228:cluster{"状态":bool, "代码":i32, "源":string})  [unwired: 8 in, 1 out]
      }
      n120 = call "CCD Loop.vi"("数据通知器"=w21, "CAM"=w20, "Director"=w25) -> ("error out"=w23:errorcluster)  [unwired: 8 in]
      n121 = while {
        shift-right: [w1542] -> w47
        shift-left: w59 -> [w1543]
        tunnel: w41 -> [w1541]
        tunnel: [w1537] -> w48
        stop <- w1538 stop-if-true
        # "UI事件产生"
        n122 = event shown="[1] \"Sample\": 值改变" {
          selector: w1543 -> [_ _ _ _ _]
          dyn-events: [_ _ _ _ _] -> w1542
          timeout: _ -> [_ _ _ _ _]
          tunnel: w1541 -> [w1546 w1550 w1554 w1555 w1557]
          tunnel: [_ w1549 w1552 w1555 w1557] -> w1540
          tunnel: [w1544 w1548 w1551 _ _] -> w1539
          tunnel: [_ _ _ _ TRUE] -> w1538
          event "停止": Value Change {
            n123 = event-data() -> ()  [unwired: 1 in, 1 out]
            n124 = call-poly "Enqueue Message.vi"("消息"="Stop", "消息队列"=w1546) -> ("error out"=w1544:cluster{"状态":bool, "代码":i32, "源":string})  [unwired: 8 in, 1 out]
          }
          event "Sample": Value Change {
            n125 = event-data() -> ()  [unwired: 1 in, 1 out]
            n126 = call-poly "Enqueue Message.vi"("消息"="Sample", "消息队列"=w1550) -> ("error out"=w1548:cluster{"状态":bool, "代码":i32, "源":string}, "消息队列副本"=w1549:refnum<queue>)  [unwired: 8 in]
          }
          event Panel Close {
            n127 = event-data() -> ()  [unwired: 1 in, 1 out]
            n128 = call-poly "Enqueue Message.vi"("消息"="Confirm Quit", "消息队列"=w1554) -> ("error out"=w1551:cluster{"状态":bool, "代码":i32, "源":string}, "消息队列副本"=w1552:refnum<queue>)  [unwired: 8 in]
          }
          event Application Instance Close {
            n129 = event-data() -> ()  [unwired: 1 in, 1 out]
          }
          event User Event {
            n130 = event-data() -> ()  [unwired: 1 in, 1 out]
          }
        }
        n131 = call "Error Handler - Event Handling Loop.vi"("error in (no error)"=w1539, "消息队列"=w1540) -> ("错误输入副本"=w1537:cluster{"状态":bool, "代码":i32, "源":string})  [unwired: 8 in, 1 out]
      }
      n132 = call "DAQ Loop.vi"("数据通知器"=w29, "DAQ"=w39, "Director"=w25) -> ("error out"=w32:errorcluster)  [unwired: 8 in]
      n133 = while {
        tunnel: w20 -> [w1219]
        stop <- w1218 stop-if-true
        # "CCD Display Loop"
        n134 = Wait on Notification(notifier=w1219) -> (notification=→"CCD Image":T2, error out=w1218:errorcluster)  [unwired: 3 in, 2 out]
        n135 = Wait (ms)(milliseconds to wait=u32 30 ("等待时间（毫秒）")) -> ()  [unwired: 1 out]
      }
      n136 = call "Logging Message Loop.vi"("数据队列"=w29, "消息队列"=w25) -> ("error out"=w27:cluster{"状态":bool, "代码":i32, "源":string})  [unwired: 9 in]
      n137 = call "CCD Log Loop.vi"("数据队列"=w21, "消息队列"=w25) -> ("error out"=w22:cluster{"状态":bool, "代码":i32, "源":string})  [unwired: 9 in]
      n138 = Merge Errors(w23, w22) -> (w24:errorcluster)
      n139 = Release Notifier(notifier=w20, error in (no error)=w24) -> (error out=w38:errorcluster)  [unwired: 1 in, 2 out]
      n140 = Release Queue(queue=w21, error in (no error)=w38) -> (error out=w30:errorcluster)  [unwired: 1 in, 2 out]
      n141 = Unregister For Events(event registration refnum=w47, error in=w48) -> (error out=w46:errorcluster)
      n142 = Release Queue(queue=w41, error in (no error)=w42) -> (error out=w33:errorcluster)  [unwired: 1 in, 2 out]
      n143 = Merge Errors(w32, w27, w28) -> (w31:errorcluster)
      n144 = Release Notifier(notifier=w39, error in (no error)=w31) -> (error out=w40:errorcluster)  [unwired: 1 in, 2 out]
      n145 = Release Queue(queue=w29, error in (no error)=w40) -> (error out=w34:errorcluster)  [unwired: 1 in, 2 out]
      n146 = Unbundle By Name(w49) -> ("hDevice"=w43:i32)
      n147 = Merge Errors(w46, w45, w33, w34, w30) -> (w44:errorcluster)
      n148 = call "USB9825_DO.vi"("Error In"=w44, "pDO"=u8 0, "hDevice"=w43) -> ("Error Out"=w63:errorcluster)  [unwired: 8 in]
      n149 = call "USB9825_AD_UnLink.vi"("Error In"=w63, "hDevice"=w43) -> ("Error Out"=w62:errorcluster)  [unwired: 9 in]
      n150 = disable-structure shown="启用" {
        disable-tunnel: w6 -> [w1560 _]
        disable-tunnel: w62 -> [w1559 w1561]
        disable-tunnel: [w1558 w1561] -> w64
        frame Disabled {
          # "调试时，启用该程序框图"
          n151 = call <vilib>:"DB Tools Close Connection.vi"("error in (no error)"=w1559, "connection reference"=w1560) -> ("error out"=w1558:errorcluster)  [unwired: 5 in]
        }
        frame Enabled {
        }
      }
    }
    frame Error {
    }
  }
  "error out" <- w1
